vi "InterpolatePoints.vi"(9 "Scaling Factor":i32, 10 "Previous Coord":cluster{"x (mm)":dbl, "y (mm)":dbl}, 11 "Current Coord":cluster{"x (mm)":dbl, "y (mm)":dbl}) -> (3 "Array":dbl[][](array[numeric]))   [LabVIEW 2024]
panel:
  in  "input variable":dbl=10.0
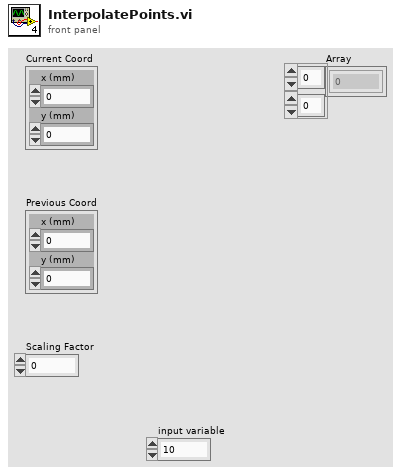
[diagram p1: front panel]
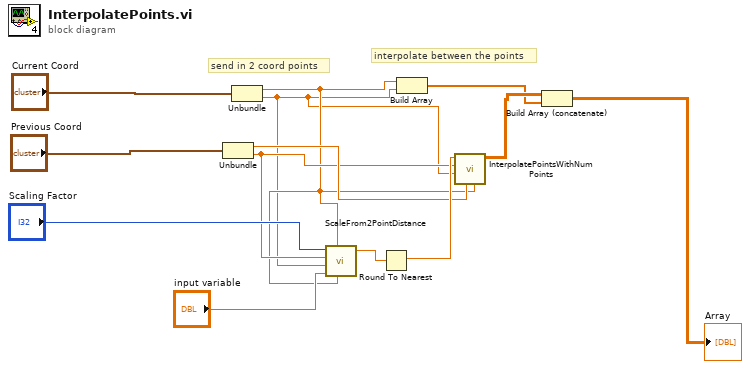
[diagram p0: block diagram]
diagram:
  # "interpolate between the points"
  # "send in 2 coord points"
  n1 = Unbundle("Previous Coord") -> ("x (mm)"=w5:dbl, "y (mm)"=w4:dbl)
  n2 = Unbundle("Current Coord") -> ("x (mm)"=w3:dbl, "y (mm)"=w2:dbl)
  n3 = call "ScaleFrom2PointDistance.vi"("x1"=w3, "x2"=w3, "k"="input variable", "y2"=w2, "y1"=w4, "Scaling Factor"="Scaling Factor") -> ("Numeric"=w9:dbl)  [unwired: 5 in]
  n4 = Round To Nearest(number=w9) -> (nearest integer value=w8:dbl)
  n5 = Build Array(w3, w2) -> (w1:dbl[])
  n6 = call "InterpolatePointsWithNumPoints.vi"("x2"=w3, "x1"=w5, "y2"=w2, "y1"=w4, "Scale # points"=w8) -> ("Array out"=w12:dbl[][])  [unwired: 6 in]
  n7 = Build Array (concatenate)(w12, w1) -> (→"Array":dbl[][])
